vi "String Matrix Is Numeric.vi"(2 "scan format (%.;%e)":string="%.;%e", 3 "string matrix":string[][](array[string])) -> (0 "numeric matrix":dbl[][](array[numeric]), 1 "is numeric":bool)   [LabVIEW 2020]
doc: "Detects if whole String matrix is pure numeric. If it contains some rubbish after or before number it will be non-numeric."
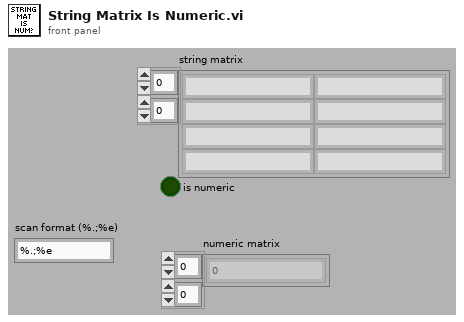
[diagram p1: front panel]
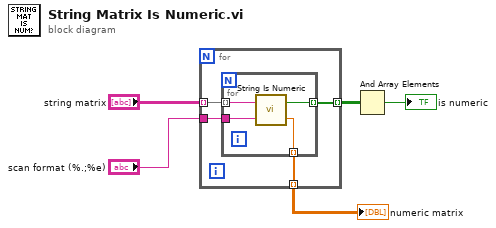
[diagram p0: block diagram]
diagram:
  n1 = for {
    tunnel: "string matrix" -> [w9] mode=indexing
    tunnel: "scan format (%.;%e)" -> [w8]
    tunnel: [w7] -> w3 mode=indexing
    tunnel: [w6] -> w1 mode=indexing
    n2 = for {
      tunnel: w9 -> [w13] mode=indexing
      tunnel: w8 -> [w12]
      tunnel: [w11] -> w7 mode=indexing
      tunnel: [w10] -> w6 mode=indexing
      n3 = call "String Is Numeric.vi"("scan format (%.;%e)"=w12, "String"=w13) -> ("Numeric"=w10:dbl, "is numeric"=w11:bool)
    }
  }
  "numeric matrix" <- w1
  n4 = And Array Elements(Boolean array=w3) -> (logical AND=→"is numeric":bool)
